vi "Altitude Only Feet.vi"() -> ()   [LabVIEW 2012]
panel:
  in  "OK Button":bool
  out "Altitude":dbl=88888.0
  # "Current Effective Latitude in Feet"
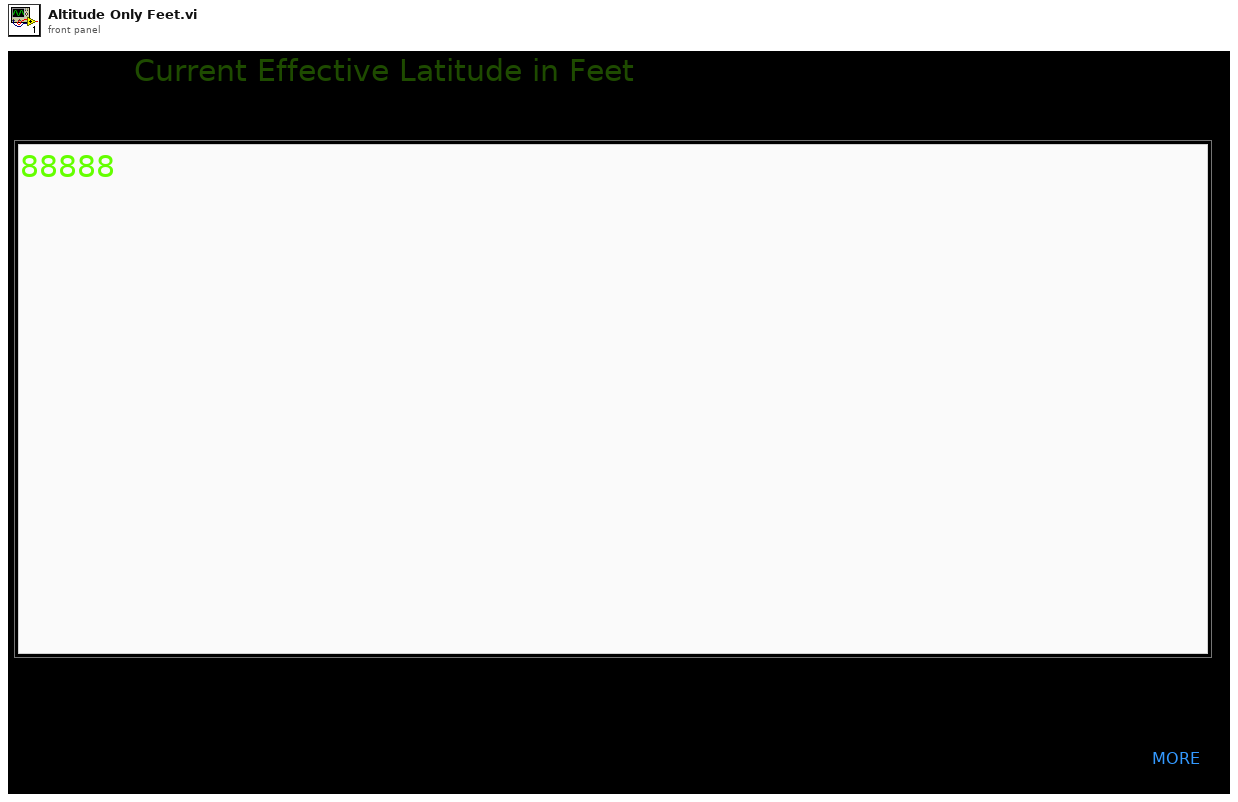
[diagram p1: front panel]
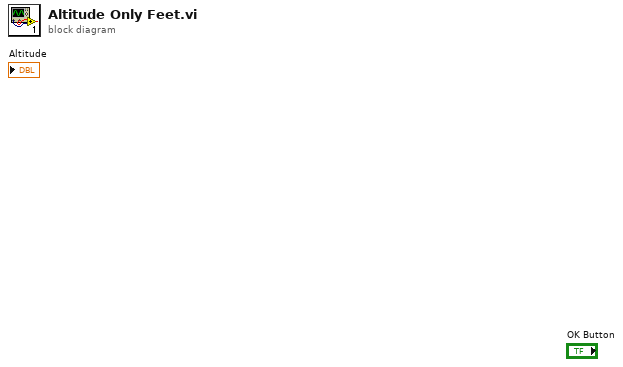
[diagram p0: block diagram]
diagram:
